vi "MaxMin.vi"() -> ()   [LabVIEW 2017]
panel:
  out "Image":T1(plugin-control)
  in  "error in (no error)":errorcluster
  out "error out":errorcluster
  out "Maximal Value":sgl
  out "Minimal Value":sgl
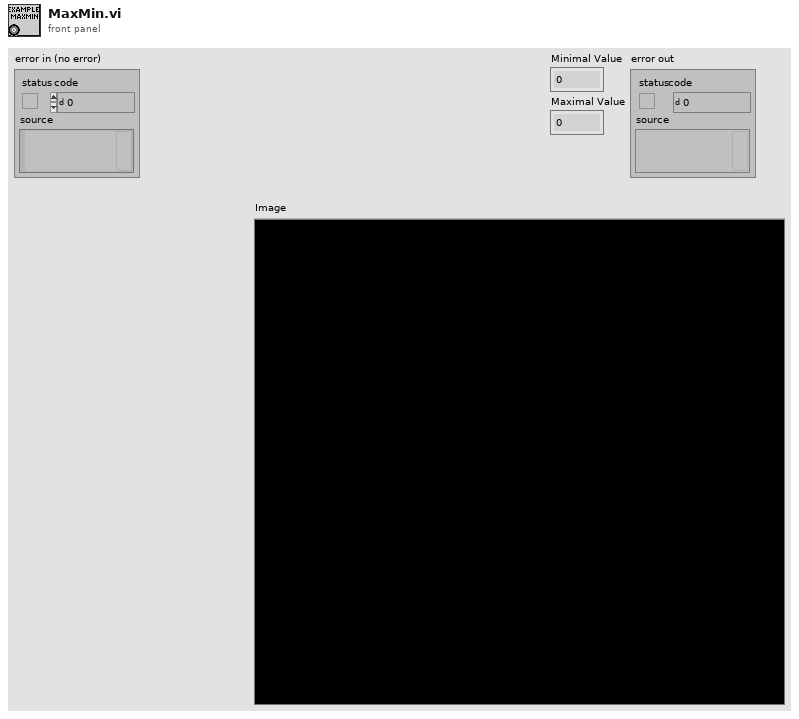
[diagram p1: front panel]
types:
  T1 = typedef "IMAQ Image.ctl" = refnum<image>
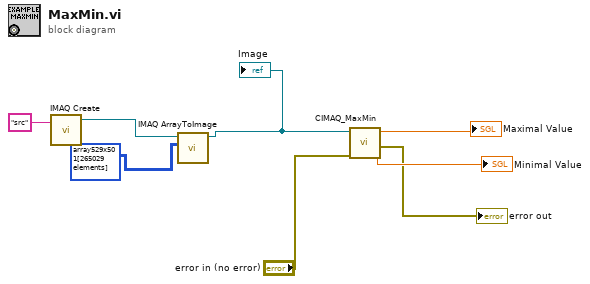
[diagram p0: block diagram]
diagram:
  n1 = call "IMAQ Create"("Image Name"="src") -> ("New Image"=w3:T1)  [unwired: 4 in, 1 out]
  n2 = call "IMAQ ArrayToImage"("Image Pixels (U8)"=u8[][] array529x501[265029 elements], "Image"=w3) -> ("Image Out"=w1:T1)  [unwired: 8 in, 1 out]
  "Image" <- w1
  n3 = call "CIMAQ_MaxMin.vi"("error in (no error)"="error in (no error)", "Img In"=w1) -> ("error out"=→"error out":errorcluster, "Minimal Value"=→"Minimal Value":sgl, "Maximal Value"=→"Maximal Value":sgl)  [unwired: 7 in]
